vi "New.vi"(6 "Configuration":string, 7 "Class Manager Reference":refnum<data-value>, 8 "error in (no error)":errorcluster, 10 "Name":string, 11 "Child Class in":refnum<class "Application.lvclass">) -> (0 "error out":errorcluster, 3 "Child Class out":refnum<class "Application.lvclass">)   [LabVIEW 2017, in "Application.lvlib" / "Application.lvclass"]
uses:
  Application.lvclass
  <vilib>/TSS/ACRObat Test Framework/Classes/Class Register/Class Register.lvclass
  <vilib>/TSS/ACRObat Test Framework/Classes/Base Objects/Base Class/Base Class/Base Class.lvclass
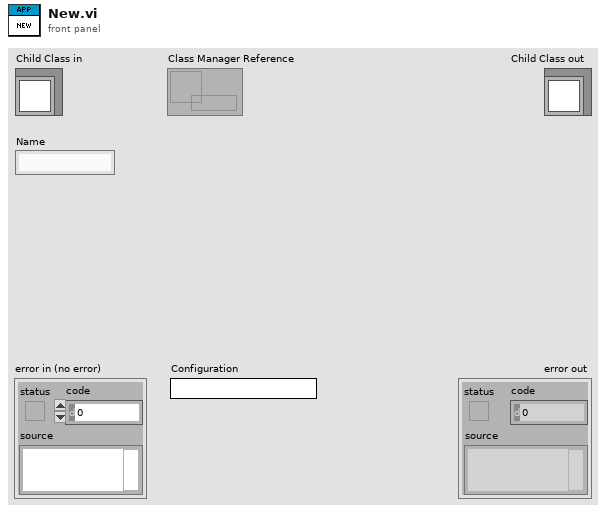
[diagram p1: front panel]
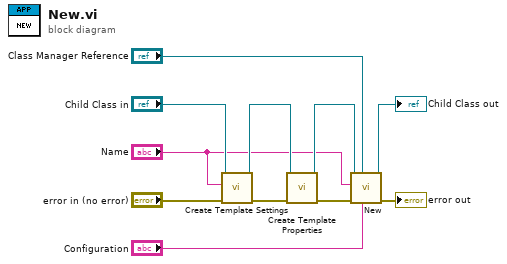
[diagram p0: block diagram]
diagram:
  n1 = call "Create Template Settings.vi"("error in (no error)"="error in (no error)", "Name"="Name", "Acrobat Template in"="Child Class in") -> ("error out"=w4:errorcluster, "Acrobat Template out"=w2:refnum<class "Application.lvclass">)  [unwired: 7 in]
  n2 = call "Create Template Properties.vi"("error in (no error)"=w4, "Acrobat Template in"=w2) -> ("error out"=w7:errorcluster, "Acrobat Template out"=w6:refnum<class "Application.lvclass">)  [unwired: 8 in]
  n3 = call-parent "New.vi"("Configuration"="Configuration", "Class Manager Reference"="Class Manager Reference", "error in (no error)"=w7, "Name"="Name", "Base Class in"=w6) -> ("error out"=→"error out":errorcluster, "Base Class out"=→"Child Class out":refnum<class "Application.lvclass">)  [unwired: 5 in]
